vi "GetFrameReferences.vi"(6 "error in":errorcluster, 9 "FlatSequence in":refnum<class "FlatSequence.lvclass">) -> (0 "error out":errorcluster, 3 "FlatSequence out":refnum<class "FlatSequence.lvclass">, 4 "Frames[]":refnum<vi>[](array[refnum]))   [LabVIEW 2014, in "FlatSequence.lvclass"]
uses:
  FlatSequence.lvclass
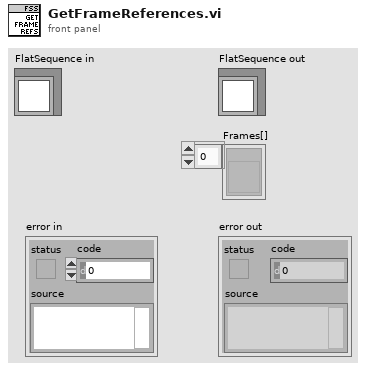
[diagram p1: front panel]
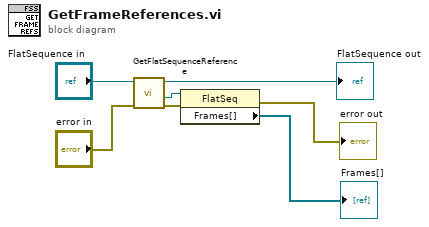
[diagram p0: block diagram]
diagram:
  n1 = call "GetFlatSequenceReference.vi"("error in"="error in", "FlatSequence in"="FlatSequence in") -> ("error out"=w4:errorcluster, "reference out"=w5:refnum<vi>, "FlatSequence out"=→"FlatSequence out":refnum<class "FlatSequence.lvclass">)  [unwired: 7 in]
  n2 = property class="FlatSeq"(reference=w5, error in=w4) -> (error out=→"error out":errorcluster, "Frames[]"=→"Frames[]":refnum<vi>[])  [unwired: 1 out]
